vi "Increment DNUM.vi"(8 "error in (no error)":errorcluster, 11 "TSM context":T1) -> (0 "error out":errorcluster, 3 "DCOUNT":i32)   [LabVIEW 2019]
uses:
  <vilib>/NI_TestStand_SemiconductorModule/NI_TestStand_Semiconductor_Module.lvlibp/PinMap/General/SemiconductorModuleContext.ctl
  TSM Context Data Access/TSM Context Data Access.lvclass/TSM Context Data Access.ctl
  TSM Context Data Access/Public/Properties/DNUM - Read.vi
  TSM Context Data Access/Public/Properties/DNUM - Write.vi
  <vilib>/NI_TestStand_SemiconductorModule/NI_TestStand_Semiconductor_Module.lvlibp/PinMap/Site and Global Data/GetGlobalData.vi
  <vilib>/NI_TestStand_SemiconductorModule/NI_TestStand_Semiconductor_Module.lvlibp/PinMap/Site and Global Data/SetGlobalData.vi
  TSM Context Data Access/TSM Context Data Access.lvclass
  <vilib>/NI_TestStand_SemiconductorModule/NI_TestStand_Semiconductor_Module.lvlibp
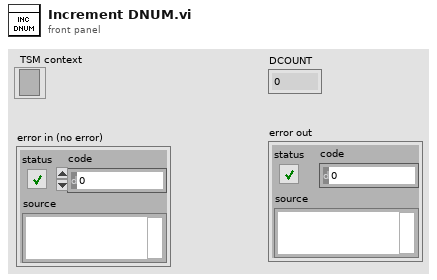
[diagram p1: front panel]
types:
  T1 = typedef "NI_TestStand_Semiconductor_Module.lvlibp/SemiconductorModuleContext.ctl" = refnum<k7>
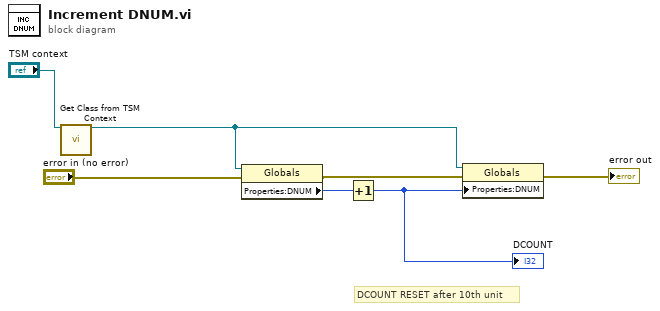
[diagram p0: block diagram]
diagram:
  # "DCOUNT RESET after 10th unit"
  n1 = call "Get Class from TSM Context.vi"("TSM Context"="TSM context") -> ("Global Memory Class"=w4:refnum<class "TSM Context Data Access.lvclass">)  [unwired: 14 in]
  n2 = property class="Globals"(reference=w4, error in="error in (no error)") -> (error out=w5:errorcluster, "Properties:DNUM"=w2:i32)  [unwired: 1 out]
  n3 = Increment(x=w2) -> (x+1=w1:i32)
  "DCOUNT" <- w1
  n4 = property class="Globals"(reference=w4, error in=w5, "Properties:DNUM"=w1) -> (error out=→"error out":errorcluster)  [unwired: 1 out]
